vi "Initialize DMD 1 Control (SubVI).vi"() -> (1 "DMD IMG REF":refnum<vi>, 2 "STOP REF":refnum<vi>, 3 "DMD VI REF":refnum<vi>)   [LabVIEW 2020]
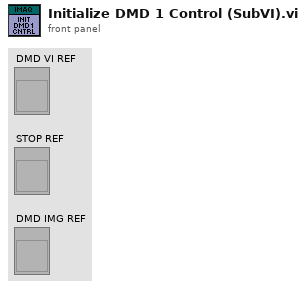
[diagram p1: front panel]
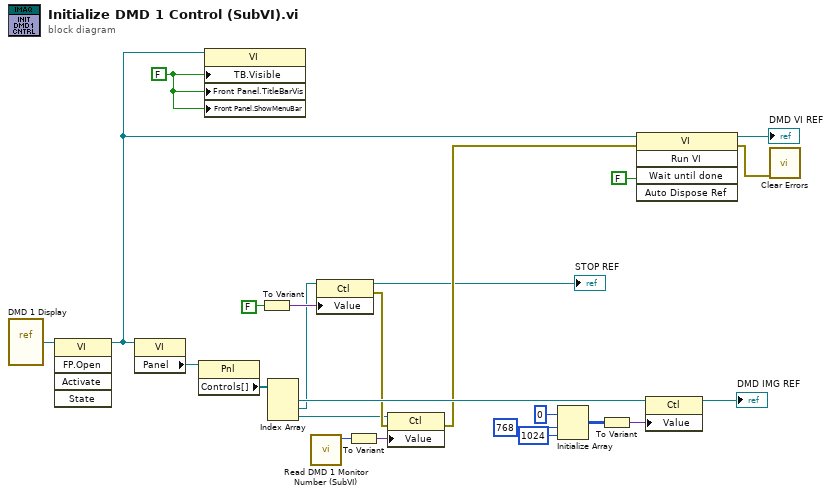
[diagram p0: block diagram]
diagram:
  w10 = FALSE ("Tool Bar:Visible")
  n1 = vi-ref "DMD 1 Display.vi"() -> (w2:refnum<vi>)
  n2 = invoke class="VI" method="FP.Open"(reference=w2) -> (reference out=w11:refnum<vi>)  [unwired: 4 in, 4 out]
  n3 = property class="VI"(reference=w11) -> ("Panel"=w5:refnum<vi>)  [unwired: 1 in, 2 out]
  n4 = property class="Pnl"(reference=w5) -> ("Controls[]"=w4:refnum<vi>[])  [unwired: 1 in, 2 out]
  n5 = property class="VI"(reference=w11, "TB.Visible"=w10, "Front Panel.TitleBarVis"=w10, "Front Panel.ShowMenuBar"=w10) -> ()  [unwired: 1 in, 2 out]
  n6 = To Variant(anything=FALSE ("Wait Until Done")) -> (Variant=w8:variant)
  n7 = Index Array(array=w4) -> (element #1=w22:refnum<vi>, element #2=w7:refnum<vi>, element #3=w13:refnum<vi>)  [unwired: 3 in]
  n8 = call "Read DMD 1 Monitor Number (SubVI).vi"() -> ("Monitor Number"=w14:u16)  [unwired: 11 in]
  n9 = property class="Ctl"(reference=w7, "Value"=w8) -> (reference out=→"STOP REF":refnum<vi>, error out=w15:errorcluster)  [unwired: 1 in]
  n10 = To Variant(anything=w14) -> (Variant=w12:variant)
  n11 = property class="Ctl"(reference=w13, error in=w15, "Value"=w12) -> (error out=w16:errorcluster)  [unwired: 1 out]
  n12 = Initialize Array(u8 0 ("element"), 768 ("dimension size"), 1024 ("dimension size")) -> (w24:u8[][])
  n13 = To Variant(anything=w24) -> (Variant=w21:variant)
  n14 = invoke class="VI" method="Run VI"(reference=w11, error in=w16, "Wait until done"=FALSE ("Wait Until Done")) -> (reference out=→"DMD VI REF":refnum<vi>, error out=w1:errorcluster)  [unwired: 2 in, 3 out]
  n15 = property class="Ctl"(reference=w22, "Value"=w21) -> (reference out=→"DMD IMG REF":refnum<vi>)  [unwired: 1 in, 1 out]
  n16 = call <vilib>:"Clear Errors.vi"("error in (no error)"=w1) -> ()  [unwired: 5 in, 2 out]
